vi "fpga_main.vi"() -> ()   [LabVIEW 2021]
doc: "This vi includes main loop on the FPGA."
uses:
  fpga_dtype_threshold.ctl
  fpga_dtype_sgl_8ch.ctl
  fpga_dtype_sgl_fb.ctl
  fpga_dtype_scan_config.ctl
  fpga_feedback_config.ctl
  fpga_dtype_index.ctl
  fpga_dtype_data.ctl
  fpga_dtype_status.ctl
  <vilib>/rvi/Emulation/niFpgaSctlEmulationGetInTimedLoop.vi
  <vilib>/rvi/Emulation/niFpgaProcessEmulError.vi
  <vilib>/rvi/Emulation/niFpgaGetClockAttributes.vi
  <vilib>/rvi/Emulation/niFpgaEmulationReportErrorSimple.vi
  <vilib>/rvi/Emulation/niFpgaCriticalErrorInLSC.vi
panel:
  in  "enable read target":bool=TRUE
  in  "tip guard position":sgl
  in  "Reset TG":bool
  in  "tip guard":T1={"ai limit (high)"={"ch 0"=inf, "ch 1"=inf, "ch 2"=inf, "ch 3"=inf, "ch 4"=inf, "ch 5"=inf, "ch 6"=inf, "ch 7"=inf}, "fb limit (hight)"={"fb 0"=inf, "fb 1"=inf}, "ai limit (low)"={"ch 0"=-inf, "ch 1"=-inf, "ch 2"=-inf, "ch 3"=-inf, "ch 4"=-inf, "ch 5"=-inf, "ch 6"=-inf, "ch 7"=-inf}, "fb limit (low)"={"fb 0"=-inf, "fb 1"=-inf}}
  out "target":T2
  in  "loop timer":u32 caption="loop count (Ticks)"
  out "max count":u32
  in  "reset max count":bool
  in  "slope":cluster{"x":sgl, "y":sgl}
  out "data":T4
  in  "index (manual)":T6
  in  "initial positions (manual)":T2
  in  "scan (manual)":bool
  in  "Abort":bool
  in  "ai gain":T2={"ch 0"=1.0, "ch 1"=1.0, "ch 2"=1.0, "ch 3"=1.0, "ch 4"=1.0, "ch 5"=1.0, "ch 6"=1.0, "ch 7"=1.0}
  in  "limit (high, 10 V)":T2={"ch 0"=10.0, "ch 1"=10.0, "ch 2"=10.0, "ch 3"=10.0, "ch 4"=10.0, "ch 5"=10.0, "ch 6"=10.0, "ch 7"=10.0}
  in  "limit (low, 10 V)":T2={"ch 0"=-10.0, "ch 1"=-10.0, "ch 2"=-10.0, "ch 3"=-10.0, "ch 4"=-10.0, "ch 5"=-10.0, "ch 6"=-10.0, "ch 7"=-10.0}
  in  "ao gain":T2={"ch 0"=1.0, "ch 1"=1.0, "ch 2"=1.0, "ch 3"=1.0, "ch 4"=1.0, "ch 5"=1.0, "ch 6"=1.0, "ch 7"=1.0}
  in  "DMA":bool
  in  "Power":bool
  in  "Feedback 1 config":T7
  in  "Feedback 0 config":T7
  in  "scan config":T8
  in  "speed":T2={"ch 0"=20.0, "ch 1"=20.0, "ch 2"=20.0, "ch 3"=20.0, "ch 4"=20.0, "ch 5"=20.0, "ch 6"=20.0, "ch 7"=20.0}
  in  "threshold":T1={"ai limit (high)"={"ch 0"=inf, "ch 1"=inf, "ch 2"=inf, "ch 3"=inf, "ch 4"=inf, "ch 5"=inf, "ch 6"=inf, "ch 7"=inf}, "fb limit (hight)"={"fb 0"=inf, "fb 1"=inf}, "ai limit (low)"={"ch 0"=-inf, "ch 1"=-inf, "ch 2"=-inf, "ch 3"=-inf, "ch 4"=-inf, "ch 5"=-inf, "ch 6"=-inf, "ch 7"=-inf}, "fb limit (low)"={"fb 0"=-inf, "fb 1"=-inf}}
  # "IO config"
  # "Scan config"
  # "Manual scan"
  # "Tip guard (TG) config"
  # "Feedback config"
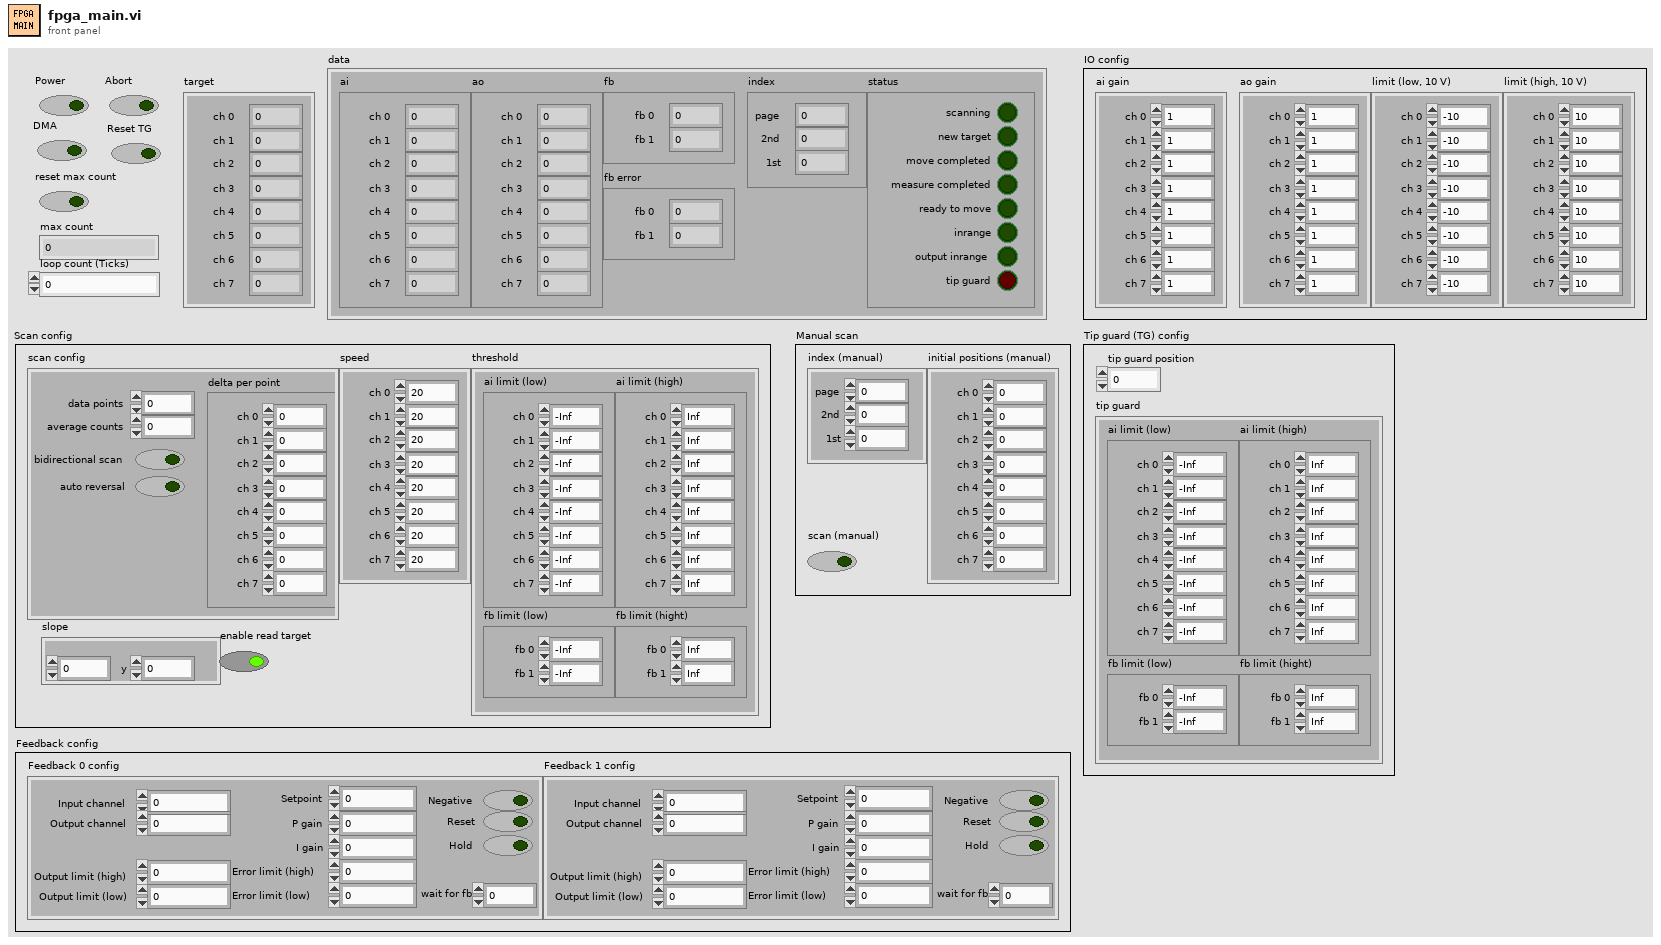
[diagram p1: front panel]
types:
  T1 = typedef "fpga_dtype_threshold.ctl" = cluster{"ai limit (high)":T2, "fb limit (hight)":T3, "ai limit (low)":T2, "fb limit (low)":T3}
  T2 = typedef "fpga_dtype_sgl_8ch.ctl" = cluster{"ch 0":sgl, "ch 1":sgl, "ch 2":sgl, "ch 3":sgl, "ch 4":sgl, "ch 5":sgl, "ch 6":sgl, "ch 7":sgl}
  T3 = typedef "fpga_dtype_sgl_fb.ctl" = cluster{"fb 0":sgl, "fb 1":sgl}
  T4 = typedef "fpga_dtype_data.ctl" = cluster{"ai":T2, "ao":T2, "fb":T3, "fb error":T3, "status":T5, "index":T6}
  T5 = typedef "fpga_dtype_status.ctl" = cluster{"scanning":bool, "new target":bool, "move completed":bool, "measure completed":bool, "inrange":bool, "ready to move":bool, "output inrange":bool, "tip guard":bool}
  T6 = typedef "fpga_dtype_index.ctl" = cluster{"page":i16, "2nd":i16, "1st":i16}
  T7 = typedef "fpga_feedback_config.ctl" = cluster{"Setpoint":sgl, "Output limit (low)":sgl, "Output limit (high)":sgl, "P gain":sgl, "I gain":sgl, "Reset":bool, "Hold":bool, "Negative":bool, "Input channel":i16, "Output channel":i16, "wait for fb":i16, "Error limit (high)":sgl, "Error limit (low)":sgl}
  T8 = typedef "fpga_dtype_scan_config.ctl" = cluster{"data points":i16, "average counts":i16, "delta per point":T2, "bidirectional scan":bool, "auto reversal":bool}
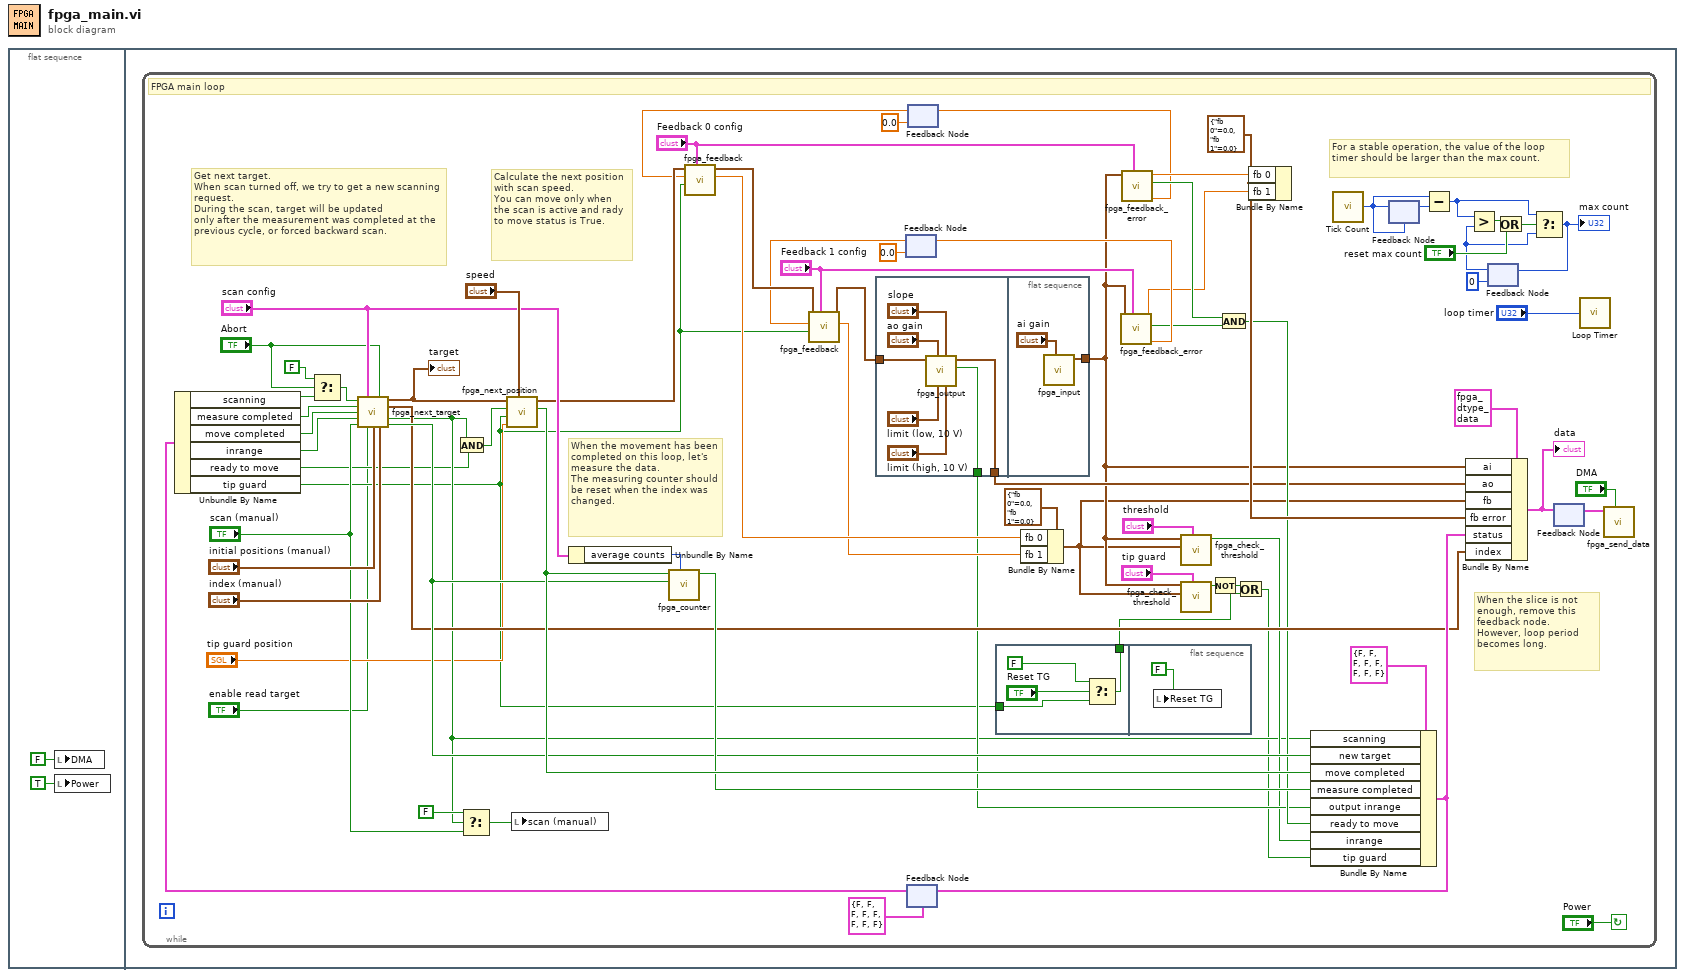
[diagram p0: block diagram]
diagram:
  n1 = flat-sequence {
    frame #0 {
      n2 = local write "DMA"(FALSE ("DMA")) -> ()
      n3 = local write "Power"(TRUE ("Power")) -> ()
    }
    frame #1 {
      n4 = while {
        stop <- "Power" continue-if-true
        w60 = T3 {"fb 0"=0.0, "fb 1"=0.0} ("sgl fb")
        # "For a stable operation, the value of the loop timer should be larger than the max count."
        # "When the slice is not enough, remove this feedback node.\nHowever, loop period becomes long."
        # "Get next target.\nWhen scan turned off, we try to get a new scanning request.\nDuring the scan, target will be updated\nonly after the measurement was completed at the previous cycle, or forced backward scan."
        # "When the movement has been completed on this loop, let's measure the data.\nThe measuring counter should be reset when the index was changed."
        # "Calculate the next position with scan speed.\nYou can move only when the scan is active and rady to move status is True."
        # "FPGA main loop"
        n5 = Unbundle By Name("scan config") -> ("average counts"=w70:i16)
        n6 = flat-sequence {
          tunnel: w61 -> [w90]
          tunnel: [w85] -> w41
          tunnel: [w84] -> w16
          tunnel: [w92] -> w12
          frame #0 {
            n7 = call "fpga_output.vi"("limit (high, 10 V)"="limit (high, 10 V)", "slope"="slope", "limit (low, 10 V)"="limit (low, 10 V)", "gain"="ao gain", "output (in)"=w90) -> ("inrange?"=w85:bool, "output (out)"=w84:T2)  [unwired: 5 in]
          }
          frame #1 {
            n8 = call "fpga_input.vi"("ai gain"="ai gain") -> ("ai"=w92:T2)  [unwired: 10 in]
          }
        }
        n9 = feedback #1(sgl 0.0 ("process variable")) -> (w50:sgl)
        n10 = feedback #2(T5 {"scanning"=FALSE, "new target"=FALSE, "move completed"=FALSE, "measure completed"=FALSE, "inrange"=FALSE, "ready to move"=FALSE, "output inrange"=FALSE, "tip guard"=FALSE} ("status")) -> (w57:T5)
        n11 = Unbundle By Name(w57) -> ("scanning"=w40:bool, "measure completed"=w72:bool, "move completed"=w14:bool, "inrange"=w36:bool, "ready to move"=w4:bool, "tip guard"=w6:bool)
        n12 = Select(t=FALSE, s="Abort", f=w40) -> (s? t:f=w39:bool)
        n13 = call "fpga_next_target.vi"("scanning"=w39, "scan config"="scan config", "abort"="Abort", "measure completed?"=w72, "move completed?"=w14, "inrange?"=w36, "scan (manual)"="scan (manual)", "Read Target"="enable read target", "initial positions (manual)"="initial positions (manual)", "index (manual)"="index (manual)") -> ("target"=w76:T2, "index"=w45:T6, "scanning"=w20:bool, "new target"=w73:bool)  [unwired: 2 in]
        "target" <- w76
        n14 = And(x=w20, y=w4) -> (x .and. y?=w67:bool)
        n15 = Select(t=FALSE, s=w20, f="scan (manual)") -> (s? t:f=w23:bool)
        n16 = call "fpga_next_position.vi"("speed"="speed", "tip guard position"="tip guard position", "tip guard?"=w6, "ready to move?"=w67, "target"=w76) -> ("move completed?"=w75:bool, "output"=w69:T2)  [unwired: 5 in]
        n17 = local write "scan (manual)"(w23) -> ()
        n18 = call "fpga_counter.vi"("max counts"=w70, "reset? (F)"=w73, "count? (T)"=w75) -> ("completed?"=w74:bool)  [unwired: 7 in, 1 out]
        n19 = feedback #3(sgl 0.0 ("process variable")) -> (w66:sgl)
        n20 = call "fpga_feedback.vi"("feedback config"="Feedback 0 config", "tip guard?"=w6, "input"=w66, "output (in)"=w69) -> ("fb out"=w65:sgl, "output (out)"=w68:T2)  [unwired: 6 in]
        n21 = call "fpga_feedback.vi"("feedback config"="Feedback 1 config", "tip guard?"=w6, "input"=w50, "output (in)"=w68) -> ("fb out"=w64:sgl, "output (out)"=w61:T2)  [unwired: 6 in]
        n22 = flat-sequence {
          tunnel: w6 -> [w81]
          tunnel: [w79] -> w5
          frame #0 {
            n23 = Select(t=FALSE, s="Reset TG", f=w81) -> (s? t:f=w79:bool)
          }
          frame #1 {
            n24 = local write "Reset TG"(FALSE ("Reset tip guard")) -> ()
          }
        }
        n25 = Bundle By Name(cluster=T3 {"fb 0"=0.0, "fb 1"=0.0} ("sgl fb"), "fb 0"=w65, "fb 1"=w64) -> (w11:T3)
        n26 = call "fpga_feedback_error.vi"("feedback config"="Feedback 1 config", "AI"=w12) -> ("process variable"=w51:sgl, "ready to move?"=w49:bool, "feedback error"=w48:sgl)  [unwired: 7 in]
        n27 = feedback-in #1(w51) -> ()
        n28 = call "fpga_feedback_error.vi"("feedback config"="Feedback 0 config", "AI"=w12) -> ("process variable"=w53:sgl, "ready to move?"=w54:bool, "feedback error"=w55:sgl)  [unwired: 7 in]
        n29 = feedback-in #3(w53) -> ()
        n30 = call "fpga_check_threshold.vi"("threshold"="threshold", "feedback"=w11, "input"=w12) -> ("inrange?"=w37:bool)  [unwired: 8 in]
        n31 = call "fpga_check_threshold.vi"("threshold"="tip guard", "feedback"=w11, "input"=w12) -> ("inrange?"=w10:bool)  [unwired: 8 in]
        n32 = Not(x=w10) -> (.not. x?=w9:bool)
        n33 = And(x=w54, y=w49) -> (x .and. y?=w42:bool)
        n34 = Or(x=w9, y=w5) -> (x .or. y?=w7:bool)
        n35 = Bundle By Name(cluster=w60, "fb 0"=w55, "fb 1"=w48) -> ()  [unwired: 1 out]
        n36 = Bundle By Name(cluster=T5 {"scanning"=FALSE, "new target"=FALSE, "move completed"=FALSE, "measure completed"=FALSE, "inrange"=FALSE, "ready to move"=FALSE, "output inrange"=FALSE, "tip guard"=FALSE} ("status"), "scanning"=w20, "new target"=w73, "move completed"=w75, "measure completed"=w74, "output inrange"=w41, "ready to move"=w42, "inrange"=w37, "tip guard"=w7) -> (w58:T5)
        n37 = feedback-in #2(w58) -> ()
        n38 = call "Tick Count"() -> ("Tick Count(Ticks)"=w32:u32)
        n39 = feedback-in #4(w32) -> ()
        n40 = feedback #4(w32) -> (w33:u32)
        n41 = Subtract(x=w32, y=w33) -> (x-y=w31:u32)
        n42 = Bundle By Name(cluster=T4 {"ai"={"ch 0"=0.0, "ch 1"=0.0, "ch 2"=0.0, "ch 3"=0.0, "ch 4"=0.0, "ch 5"=0.0, "ch 6"=0.0, "ch 7"=0.0}, "ao"={"ch 0"=0.0, "ch 1"=0.0, "ch 2"=0.0, "ch 3"=0.0, "ch 4"=0.0, "ch 5"=0.0, "ch 6"=0.0, "ch 7"=0.0}, "fb"={"fb 0"=0.0, "fb 1"=0.0}, "fb error"={"fb 0"=0.0, "fb 1"=0.0}, "status"={"scanning"=FALSE, "new target"=FALSE, "move completed"=FALSE, "measure completed"=FALSE, "inrange"=FALSE, "ready to move"=FALSE, "output inrange"=FALSE, "tip guard"=FALSE}, "index"={"page"=0, "2nd"=0, "1st"=0}} ("data"), "ai"=w12, "ao"=w16, "fb"=w11, "fb error"=w60, "status"=w58, "index"=w45) -> (w47:T4)
        "data" <- w47
        n43 = feedback #5(u32 0) -> (w24:u32)
        n44 = Greater?(x=w31, y=w24) -> (0:w30:bool)
        n45 = Or(x=w30, y="reset max count") -> (x .or. y?=w29:bool)
        n46 = Select(t=w31, s=w29, f=w24) -> (s? t:f=w27:u32)
        "max count" <- w27
        n47 = feedback-in #5(w27) -> ()
        n48 = feedback #6() -> (w46:T4)  [unwired: 1 in]
        n49 = feedback-in #6(w47) -> ()
        n50 = call "Loop Timer"("Count(Ticks)"="loop timer") -> ()  [unwired: 1 out]
        n51 = call "fpga_send_data.vi"("DMA"="DMA", "data"=w46) -> ()  [unwired: 10 in]
      }
    }
  }
